vi "NMEA_ParseMessage-GPRMC.vi"(9 "Error In":errorcluster, 10 "$GPRMC-message_IN":string) -> (1 "Error Out":errorcluster, 2 "$GPRMC-message_OUT":T1={"TimeStamp"=timestamp(0 s since 1904-01-01), "Validity"=FALSE, "Latitude"=0.0, "Latitude-Direction"=enum."North", "Longitude"=0.0, "Longitude-Direction"=enum."East", "Speed in knots"=0.0, "True course"=0.0, "Date Stamp"=timestamp(0 s since 1904-01-01), "Magnetic Variation (East/West)"=0.0} {"Magnetic Variation (East/West)" format="%.02f [deg]"; "Date Stamp" format="%<%x>T"; "True course" format="%.02f [deg]"; "Speed in knots" format="%.02f [kts]"; "Longitude" format="%0.4f [long]"; "Latitude" format="%.04f [lat]"; "TimeStamp" format="%<%.2X>T"})   [LabVIEW 2016, in "AIRMAR WeatherCaster.lvlib"]
doc: "<B>GPRMC</B>\nRecommended minimum specific GPS/Transit data"
uses:
  AIRMAR WeatherCaster.lvlib
  NMEA_GPRMC-data.ctl
  NMEA_LatitudeDirection.ctl
  NMEA_LongitudeDirection.ctl
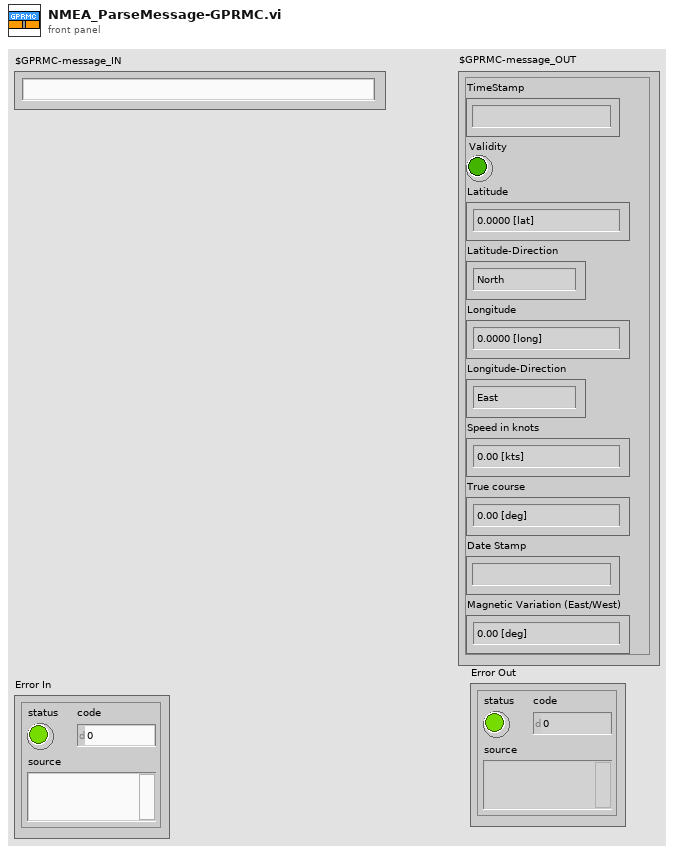
[diagram p1: front panel]
types:
  T1 = typedef "AIRMAR WeatherCaster.lvlib/NMEA_GPRMC-data.ctl" = cluster{"TimeStamp":timestamp, "Validity":bool, "Latitude":dbl, "Latitude-Direction":T2, "Longitude":dbl, "Longitude-Direction":T3, "Speed in knots":dbl, "True course":dbl, "Date Stamp":timestamp, "Magnetic Variation (East/West)":dbl}
  T2 = typedef "AIRMAR WeatherCaster.lvlib/NMEA_LatitudeDirection.ctl" = enum16{"", "North", "South"}
  T3 = typedef "AIRMAR WeatherCaster.lvlib/NMEA_LongitudeDirection.ctl" = enum16{"", "East", "West"}
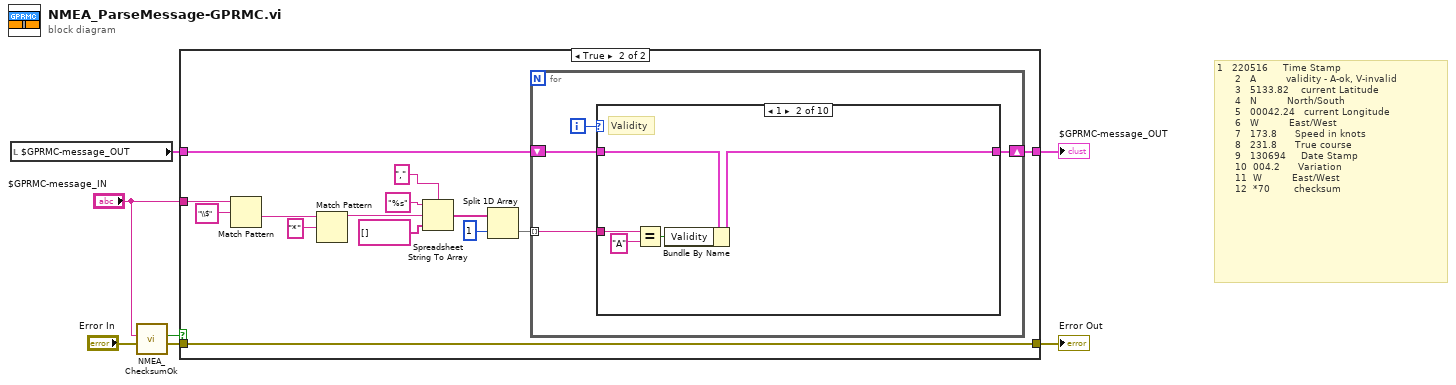
[diagram p0: block diagram]
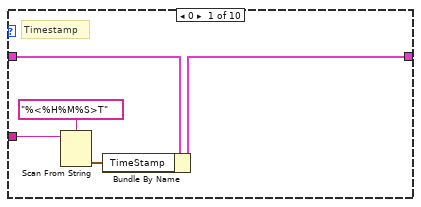
[diagram p3: hidden frame]
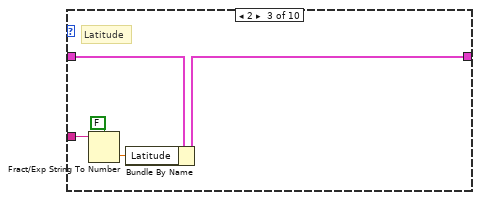
[diagram p4: hidden frame]
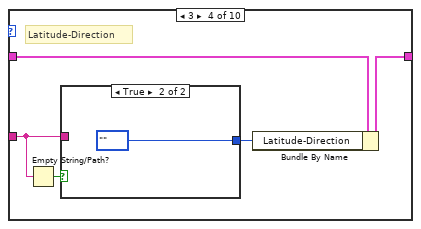
[diagram p5: hidden frame]
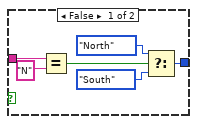
[diagram p6: hidden frame]
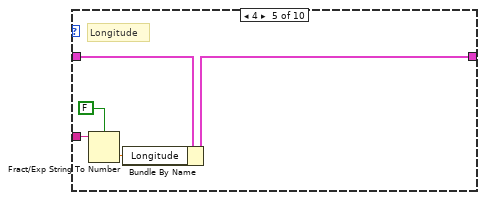
[diagram p7: hidden frame]
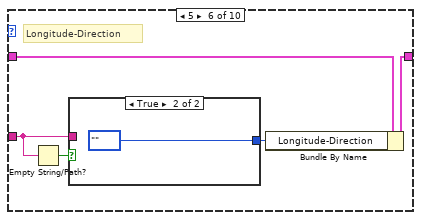
[diagram p8: hidden frame]
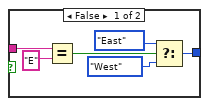
[diagram p9: hidden frame]
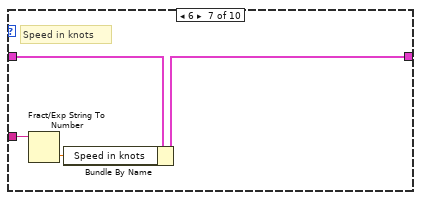
[diagram p10: hidden frame]
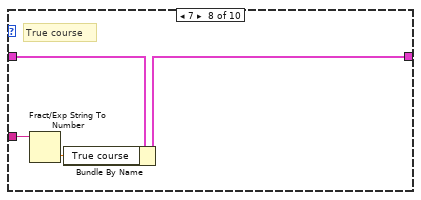
[diagram p11: hidden frame]
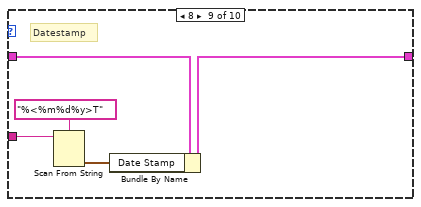
[diagram p12: hidden frame]
diagram:
  # "1   220516     Time Stamp\n      2   A          validity - A-ok, V-invalid\n      3   5133.82    current Latitude\n      4   N          North/South\n      5   00042.24   current Longitude\n      6   W          East/West\n      7   173.8      Speed in knots\n      8   231.8      True course\n      9   130694     Date Stamp\n      10  004.2      Variation\n      11  W          East/West\n      12  *70        checksum"
  n1 = local read "$GPRMC-message_OUT"() -> (w7:T1)
  n2 = call "NMEA_ChecksumOk.vi"("Error In"="Error In", "Sentence"="$GPRMC-message_IN") -> ("Error Out"=w1:errorcluster, "CheckSumOk?"=w4:bool)  [unwired: 8 in]
  n3 = case shown="True" w4 {
    tunnel: w7 -> [w9 w18]
    tunnel: [w9 w17] -> w6
    tunnel: "$GPRMC-message_IN" -> [_ w15]
    tunnel: w1 -> [w8 w10]
    tunnel: [w8 w10] -> w3
    frame False {
    }
    frame True {
      n4 = Match Pattern(string=w15, regular expression="\\$") -> (after substring=w14:string)  [unwired: 1 in, 3 out]
      n5 = Match Pattern(string=w14, regular expression="*") -> (before substring=w22:string)  [unwired: 1 in, 3 out]
      n6 = Spreadsheet String To Array(delimiter (Tab)=",", format string="%s", spreadsheet string=w22, array type (2D Dbl)=string[] []) -> (array=w12:string[])
      n7 = Split 1D Array(array=w12, index=1) -> (second subarray=w13:string[])  [unwired: 1 out]
      n8 = for {
        tunnel: w13 -> [w24] mode=indexing
        shift-right: [w26] -> w17
        shift-left: w18 -> [w27]
        i -> [w25]
        n9 = case shown="1" w25 {
          tunnel: w27 -> [w32 w37 w42 w47 w59 w64 w75 w79 w84 w85]
          tunnel: [w31 w36 w41 w46 w58 w63 w74 w78 w83 w85] -> w26
          tunnel: w24 -> [w29 w35 w40 w44 w57 w61 w73 w77 w81 _]
          frame 0 {
            # "Timestamp"
            n10 = Scan From String(format string="%<%H%M%S>T", input string=w29) -> (output 1=w28:timestamp)  [unwired: 3 in, 3 out]
            n11 = Bundle By Name(cluster=w32, "TimeStamp"=w28) -> (w31:T1)
          }
          frame 1 {
            # "Validity"
            n12 = Equal?(x=w35, y="A") -> (x = y?=w33:bool)
            n13 = Bundle By Name(cluster=w37, "Validity"=w33) -> (w36:T1)
          }
          frame 2 {
            # "Latitude"
            n14 = Fract/Exp String To Number(use system decimal point (T)=FALSE, string=w40) -> (number=w39:dbl)  [unwired: 2 in, 1 out]
            n15 = Bundle By Name(cluster=w42, "Latitude"=w39) -> (w41:T1)
          }
          frame 3 {
            # "Latitude-Direction"
            n16 = Empty String/Path?(string/path=w44) -> (empty?=w43:bool)
            n17 = case shown="True" w43 {
              tunnel: [w50 NMEA_LatitudeDirection."" ("f")] -> w45
              tunnel: w44 -> [w48 _]
              frame False {
                n18 = Equal?(x=w48, y="N") -> (x = y?=w52:bool)
                n19 = Select(t=NMEA_LatitudeDirection."North" ("Latitude-Direction"), s=w52, f=NMEA_LatitudeDirection."South") -> (s? t:f=w50:T2)
              }
              frame True {
              }
            }
            n20 = Bundle By Name(cluster=w47, "Latitude-Direction"=w45) -> (w46:T1)
          }
          frame 4 {
            # "Longitude"
            n21 = Fract/Exp String To Number(use system decimal point (T)=FALSE, string=w57) -> (number=w56:dbl)  [unwired: 2 in, 1 out]
            n22 = Bundle By Name(cluster=w59, "Longitude"=w56) -> (w58:T1)
          }
          frame 5 {
            # "Longitude-Direction"
            n23 = Empty String/Path?(string/path=w61) -> (empty?=w60:bool)
            n24 = case shown="True" w60 {
              tunnel: w61 -> [w70 _]
              tunnel: [w66 NMEA_LongitudeDirection."" ("f")] -> w62
              frame False {
                n25 = Equal?(x=w70, y="E") -> (x = y?=w68:bool)
                n26 = Select(t=NMEA_LongitudeDirection."East" ("Longitude-Direction"), s=w68, f=NMEA_LongitudeDirection."West") -> (s? t:f=w66:T3)
              }
              frame True {
              }
            }
            n27 = Bundle By Name(cluster=w64, "Longitude-Direction"=w62) -> (w63:T1)
          }
          frame 6 {
            # "Speed in knots"
            n28 = Fract/Exp String To Number(string=w73) -> (number=w72:dbl)  [unwired: 3 in, 1 out]
            n29 = Bundle By Name(cluster=w75, "Speed in knots"=w72) -> (w74:T1)
          }
          frame 7 {
            # "True course"
            n30 = Fract/Exp String To Number(string=w77) -> (number=w76:dbl)  [unwired: 3 in, 1 out]
            n31 = Bundle By Name(cluster=w79, "True course"=w76) -> (w78:T1)
          }
          frame 8 {
            # "Datestamp"
            n32 = Scan From String(format string="%<%m%d%y>T", input string=w81) -> (output 1=w80:timestamp)  [unwired: 3 in, 3 out]
            n33 = Bundle By Name(cluster=w84, "Date Stamp"=w80) -> (w83:T1)
          }
          frame Default {
          }
        }
      }
    }
  }
  "$GPRMC-message_OUT" <- w6
  "Error Out" <- w3
